vi "Keyence.Cmd.FocusAdjustment.vi"(6 "Timeout [ms] (1000)":i32=1000, 8 "error in":errorcluster, 11 "cID in":refnum<k5>) -> (0 "error out":errorcluster, 1 "OK?":bool, 2 "Response":string, 3 "cID out":refnum<k5>)   [LabVIEW 2016]
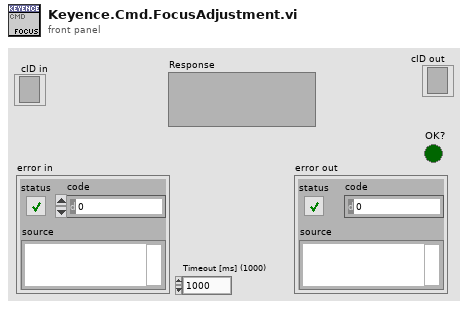
[diagram p1: front panel]
types:
  T1 = enum16{"Standard", "Buffered", "CRLF", "Immediate"}
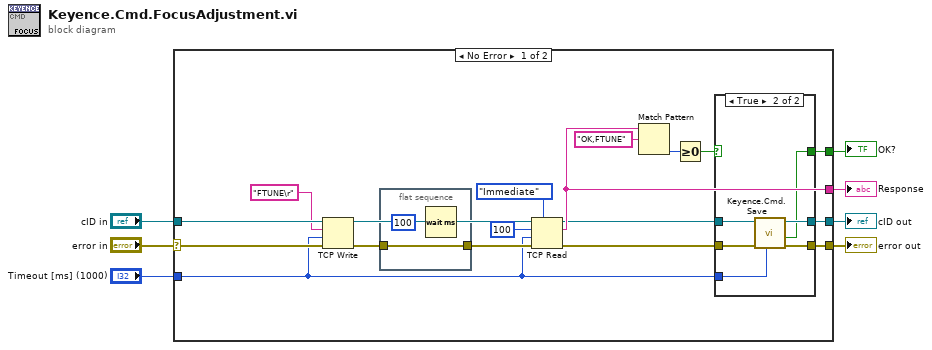
[diagram p0: block diagram]
diagram:
  n1 = case shown="No Error" "error in" {
    selector: "error in" -> [w21 w37]
    tunnel: "Timeout [ms] (1000)" -> [w9 _]
    tunnel: "cID in" -> [w22 w38]
    tunnel: [w12 w38] -> w4
    tunnel: [w13 w37] -> w3
    tunnel: [w11 _] -> w2
    tunnel: [w16 _] -> w1
    frame No Error {
      n2 = TCP Write(connection ID=w22, data in="FTUNE\r", error in (no error)=w21, 9:w9) -> (connection ID out=w23:refnum<k5>, error out=w25:errorcluster)  [unwired: 1 out]
      n3 = flat-sequence {
        tunnel: w25 -> [w36]
        tunnel: [w36] -> w24
        frame #0 {
          n4 = Wait (ms)(milliseconds to wait=u32 100) -> ()  [unwired: 1 out]
        }
      }
      n5 = TCP Read(connection ID=w23, bytes to read=100, error in (no error)=w24, 7:T1."Immediate" ("mode (standard)"), 9:w9) -> (connection ID out=w15:refnum<k5>, data out=w16:string, error out=w14:errorcluster)
      n6 = Match Pattern(string=w16, regular expression="OK,FTUNE") -> (offset past match=w17:i32)  [unwired: 1 in, 3 out]
      n7 = Greater Or Equal To 0?(x=w17) -> (x >= 0?=w10:bool)
      n8 = case shown="True" w10 {
        selector: w10 -> [w28 _]
        tunnel: w15 -> [w27 w34]
        tunnel: w14 -> [w26 w33]
        tunnel: [w26 w32] -> w13
        tunnel: [w27 w31] -> w12
        tunnel: [w28 w30] -> w11
        tunnel: w9 -> [_ w29]
        frame False {
        }
        frame True {
          n9 = call "Keyence.Cmd.Save.vi"("Timeout [ms] (1000)"=w29, "error in"=w33, "cID in"=w34) -> ("error out"=w32:errorcluster, "OK?"=w30:bool, "cID out"=w31:refnum<k5>)  [unwired: 6 in]
        }
      }
    }
    frame Error {
    }
  }
  "cID out" <- w4
  "Response" <- w1
  "OK?" <- w2
  "error out" <- w3
